vi "HTTP Message Analysis.vi"(11 "异步调用线程簇输入":T1) -> (3 "异步调用线程簇输出":T1)   [LabVIEW 2019, in "HTTP Server.lvlib"]
uses:
  HTTP Server.lvlib
  Async Thread.ctl
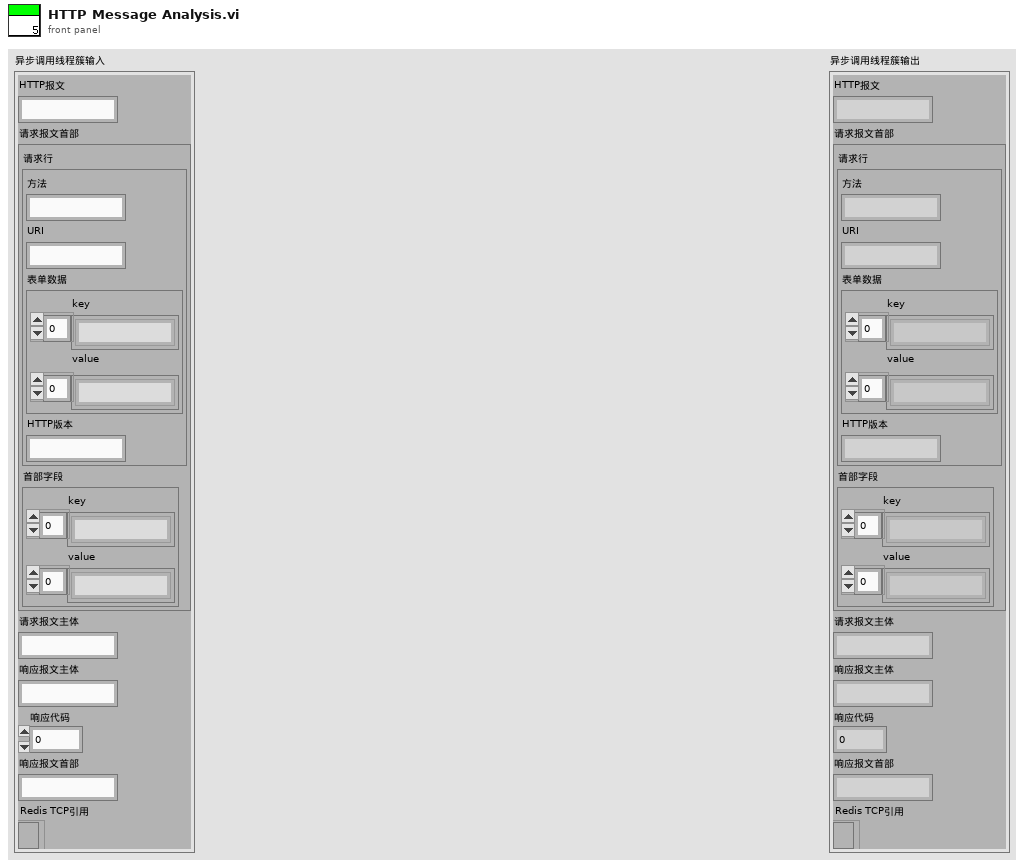
[diagram p1: front panel]
types:
  T1 = typedef "HTTP Server.lvlib/Async Thread.ctl" = cluster{"HTTP报文":string, "请求报文首部":cluster{"请求行":cluster{"方法":string, "URI":string, "表单数据":cluster{"key":string[], "value":string[]}, "HTTP版本":string}, "首部字段":cluster{"key":string[], "value":string[]}}, "请求报文主体":string, "响应报文主体":string, "响应代码":u16, "响应报文首部":string, "Redis TCP引用":refnum<k5>}
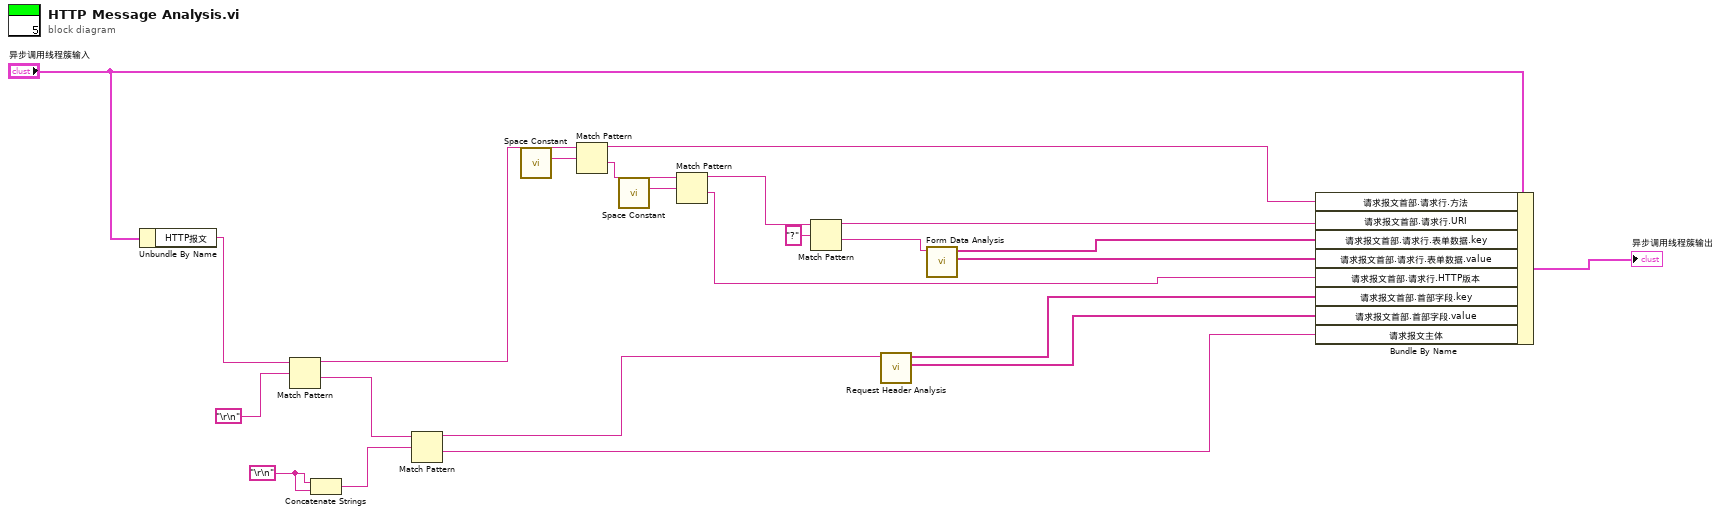
[diagram p0: block diagram]
diagram:
  w23 = "\r\n"
  n1 = Unbundle By Name("异步调用线程簇输入") -> ("HTTP报文"=w2:string)
  n2 = Match Pattern(string=w2, regular expression="\r\n") -> (before substring=w16:string, after substring=w20:string)  [unwired: 1 in, 2 out]
  n3 = Concatenate Strings(w23, w23) -> (w21:string)
  n4 = Match Pattern(string=w20, regular expression=w21) -> (before substring=w6:string, after substring=w1:string)  [unwired: 1 in, 2 out]
  n5 = call <vilib>:"Space Constant.vi"() -> ("String"=w19:string)
  n6 = Match Pattern(string=w16, regular expression=w19) -> (before substring=w17:string, after substring=w15:string)  [unwired: 1 in, 2 out]
  n7 = call <vilib>:"Space Constant.vi"() -> ("String"=w14:string)
  n8 = Match Pattern(string=w15, regular expression=w14) -> (before substring=w13:string, after substring=w7:string)  [unwired: 1 in, 2 out]
  n9 = Match Pattern(string=w13, regular expression="?" ("正则表达式")) -> (before substring=w11:string, after substring=w10:string)  [unwired: 1 in, 2 out]
  n10 = call "Request Header Analysis.vi"("请求首部字段"=w6) -> ("value"=w4:string[], "key"=w5:string[])  [unwired: 9 in]
  n11 = call "Form Data Analysis.vi"("表单数据"=w10) -> ("value"=w8:string[], "key"=w9:string[])  [unwired: 9 in]
  n12 = Bundle By Name(cluster="异步调用线程簇输入", "请求报文首部.请求行.方法"=w17, "请求报文首部.请求行.URI"=w11, "请求报文首部.请求行.表单数据.key"=w9, "请求报文首部.请求行.表单数据.value"=w8, "请求报文首部.请求行.HTTP版本"=w7, "请求报文首部.首部字段.key"=w5, "请求报文首部.首部字段.value"=w4, "请求报文主体"=w1) -> (→"异步调用线程簇输出":T1)
